vi "SetGain.vi"(8 "error in (no error)":errorcluster, 10 "Setting.Gain":i32, 11 "Camera_Prime95B in":refnum<class "Camera_Prime95B.lvclass">) -> (0 "error out":errorcluster, 3 "Camera_Prime95B out":refnum<class "Camera_Prime95B.lvclass">)   [LabVIEW 2020, in "Camera_Prime95B.lvlib" / "Camera_Prime95B.lvclass"]
uses:
  Camera_Prime95B.lvclass
  Camera_Prime95B.lvclass/Camera_Prime95B.ctl
  D:/Daguan/Development/MMicroscopyFramework/Model/Hardware Layer/Real Hardware/Camera_Prime95B/Camera_Prime95B/Dependencies/PVCamNET.dll
  Dependencies/PVCamNET.dll
  Hardware Abstraction Layer/Component/Camera/Camera/Camera.lvclass
panel:
  out "Name":string
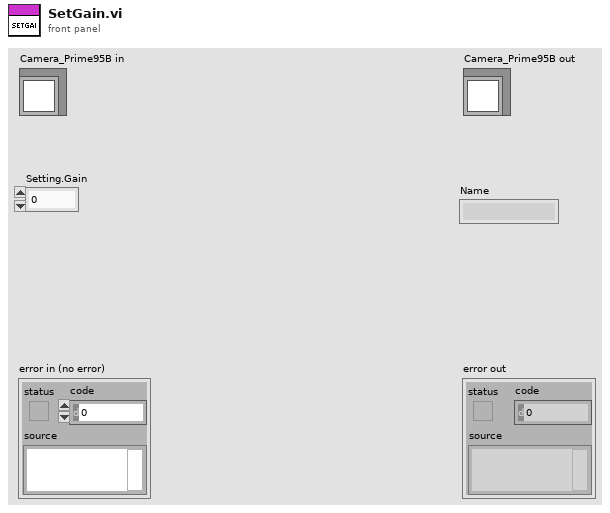
[diagram p1: front panel]
types:
  T1 = typedef "Device.lvlib/DeviceStatus.ctl" = i32
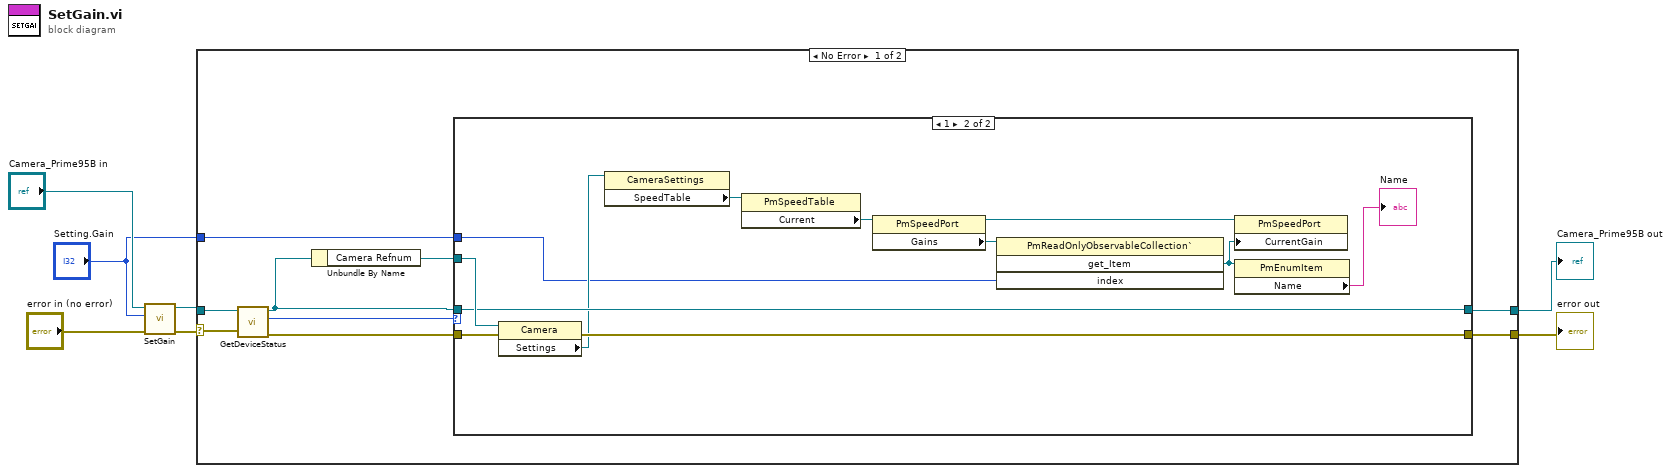
[diagram p0: block diagram]
diagram:
  n1 = call-parent "SetGain.vi"("error in (no error)"="error in (no error)", "Setting.Gain"="Setting.Gain", "Camera in"="Camera_Prime95B in") -> ("error out"=w5:errorcluster, "Camera out"=w4:refnum<class "Camera_Prime95B.lvclass">)  [unwired: 7 in]
  n2 = case shown="No Error" w5 {
    selector: w5 -> [w15 w32]
    tunnel: [w16 w32] -> w2
    tunnel: [w10 w31] -> w3
    tunnel: w4 -> [w9 w31]
    tunnel: "Setting.Gain" -> [w8 _]
    frame No Error {
      n3 = call-dynamic "GetDeviceStatus.vi"("error in (no error)"=w15, "Camera_Prime95B in"=w9) -> ("error out"=w13:errorcluster, "Status"=w14:T1, "Camera_Prime95B out"=w11:refnum<class "Camera_Prime95B.lvclass">)  [unwired: 7 in]
      n4 = Unbundle By Name(w11) -> ("Camera Refnum"=w12:refnum<k24>)
      n5 = case shown="1" w14 {
        tunnel: [w17 w30] -> w16
        tunnel: w12 -> [_ w29]
        tunnel: w13 -> [w17 w28]
        tunnel: w11 -> [w18 w27]
        tunnel: [w18 w27] -> w10
        tunnel: w8 -> [_ w20]
        frame 0, Default {
        }
        frame 1 {
          n6 = property class="Camera"(reference=w29, error in=w28) -> (error out=w30:errorcluster, "Settings"=w21:refnum<k24>)  [unwired: 1 out]
          n7 = property class="CameraSettings"(reference=w21) -> ("SpeedTable"=w26:refnum<k24>)  [unwired: 1 in, 2 out]
          n8 = property class="PmSpeedTable"(reference=w26) -> ("Current"=w23:refnum<k24>)  [unwired: 1 in, 2 out]
          n9 = property class="PmSpeedPort"(reference=w23) -> (reference out=w24:refnum<k24>, "Gains"=w22:refnum<k24>)  [unwired: 1 in, 1 out]
          n10 = invoke class="PmReadOnlyObservableCollection`" method="get_Item"(reference=w22, "index"=w20) -> ("get_Item"=w25:refnum<k24>)  [unwired: 2 in, 3 out]
          n11 = property class="PmSpeedPort"(reference=w24, "CurrentGain"=w25) -> ()  [unwired: 1 in, 2 out]
          n12 = property class="PmEnumItem"(reference=w25) -> ("Name"=→"Name":string)  [unwired: 1 in, 2 out]
        }
      }
    }
    frame Error {
    }
  }
  "error out" <- w2
  "Camera_Prime95B out" <- w3
